vi "FL_Calculate_phi_theta_etc.vi"(5 "Mouse face dir. swap":bool, 6 "x1-x2":sgl, 7 "R from center":sgl, 8 "y1-y2":sgl, 9 "Mouse Yc":sgl, 10 "MouseXc":sgl, 11 "sin(a)":sgl) -> (3 "Output data cluster":T1)   [LabVIEW 2018, in "Tracker.lvlib"]
uses:
  Tracker.lvlib
panel:
  out "Mouse rot. angle":sgl
  out "from center towards mouse":sgl
  out "Rel Y":sgl
  out "Rel X":sgl
  out "mouse wall angle":sgl
  out "phi":sgl
  out "Cage rotation against mouse":sgl
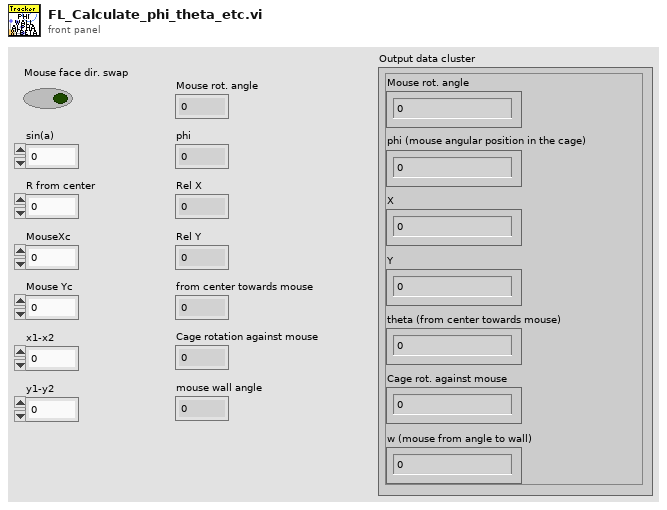
[diagram p1: front panel]
types:
  T1 = cluster{"Mouse rot. angle":sgl, "phi (mouse angular position in the cage)":dbl, "X":dbl, "Y":dbl, "theta (from center towards mouse)":dbl, "Cage rot. against mouse":sgl, "w (mouse from angle to wall)":dbl}
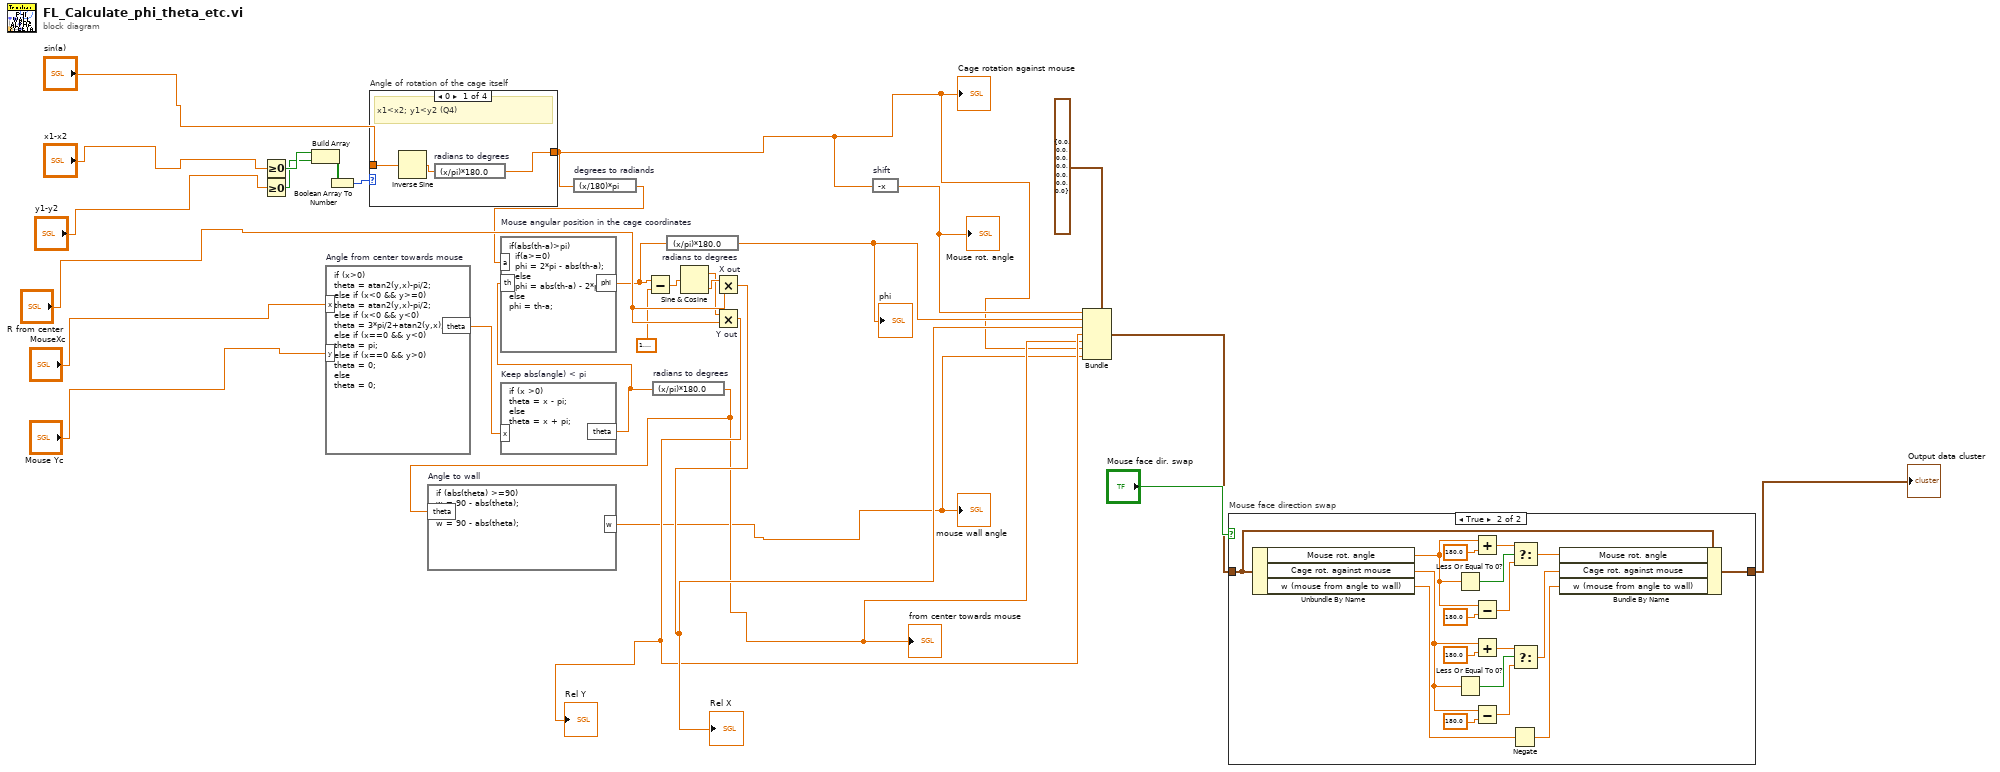
[diagram p0: block diagram]
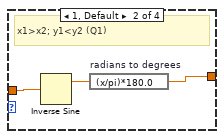
[diagram p3: hidden frame]
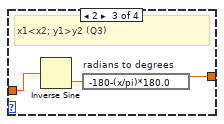
[diagram p4: hidden frame]
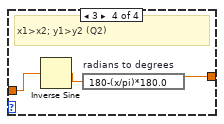
[diagram p5: hidden frame]
diagram:
  n1 = Greater Or Equal To 0?(x="x1-x2") -> (x >= 0?=w23:bool)
  n2 = Greater Or Equal To 0?(x="y1-y2") -> (x >= 0?=w22:bool)
  n3 = Build Array(w23, w22) -> (w21:bool[])
  n4 = formula code="if (x>0)\ntheta = atan2(y,x)-pi/2;\nelse if (x<0 && y>=0)\ntheta = atan2(y,x)-pi/2;\nelse if (x<0 && y<0)\ntheta = 3*pi/2+atan2(y,x);\nelse if (x==0 && y<0)\ntheta = pi;\nelse if (x==0 && y>0)\ntheta = 0;\nelse\ntheta = 0;" "Angle from center towards mouse"("x"="MouseXc", "y"="Mouse Yc") -> ("theta"=w19:dbl)
  n5 = Boolean Array To Number(Boolean array=w21) -> (number=w20:u32)
  n6 = case "Angle of rotation of the cage itself" shown="0" w20 {
    tunnel: "sin(a)" -> [w31 w34 w37 w40]
    tunnel: [w30 w33 w36 w39] -> w6
    frame 0 {
      # "x1<x2; y1<y2 (Q4)"
      n7 = Inverse Sine(1:w31) -> (0:w32:sgl)
      n8 = expression code="(x/pi)*180.0" "radians to degrees"(w32) -> (w30:sgl)
    }
    frame 1, Default {
      # "x1>x2; y1<y2 (Q1)"
      n9 = Inverse Sine(1:w34) -> (0:w35:sgl)
      n10 = expression code="(x/pi)*180.0" "radians to degrees"(w35) -> (w33:sgl)
    }
    frame 2 {
      # "x1<x2; y1>y2 (Q3)"
      n11 = Inverse Sine(1:w37) -> (0:w38:sgl)
      n12 = expression code="-180-(x/pi)*180.0" "radians to degrees"(w38) -> (w36:sgl)
    }
    frame 3 {
      # "x1>x2; y1>y2 (Q2)"
      n13 = Inverse Sine(1:w40) -> (0:w41:sgl)
      n14 = expression code="180-(x/pi)*180.0" "radians to degrees"(w41) -> (w39:sgl)
    }
  }
  "Cage rotation against mouse" <- w6
  n15 = formula code="if (x >0)\ntheta = x - pi;\nelse\ntheta = x + pi;" "Keep abs(angle) < pi"("x"=w19) -> ("theta"=w16:dbl)
  n16 = expression code="(x/180)*pi" "degrees to radiands"(w6) -> (w15:sgl)
  n17 = formula code="if(abs(th-a)>pi)\n  if(a>=0)\n  phi = 2*pi - abs(th-a);\n  else\n  phi = abs(th-a) - 2*pi;\nelse\nphi = th-a;" "Mouse angular position in the cage coordinates"("th"=w16, "a"=w15) -> ("phi"=w13:dbl)
  n18 = Subtract(x=w13, y=1.5707963267948966) -> (x-y=w14:dbl)
  n19 = expression code="(x/pi)*180.0" "radians to degrees"(w16) -> (w7:dbl)
  "from center towards mouse" <- w7
  n20 = formula code="if (abs(theta) >=90)\nw = 90 - abs(theta);\nelse\nw = 90 - abs(theta);" "Angle to wall"("theta"=w7) -> ("w"=w1:dbl)
  "mouse wall angle" <- w1
  n21 = expression code="(x/pi)*180.0" "radians to degrees"(w13) -> (w10:dbl)
  "phi" <- w10
  n22 = Sine & Cosine(0:w14) -> (1:w17:dbl, 2:w18:dbl)
  n23 = Multiply "X out"(x=w18, y="R from center") -> (x*y=w9:dbl)
  "Rel X" <- w9
  n24 = Multiply "Y out"(x=w17, y="R from center") -> (x*y=w8:dbl)
  "Rel Y" <- w8
  n25 = expression code="-x" "shift"(w6) -> (w11:sgl)
  "Mouse rot. angle" <- w11
  n26 = Bundle(cluster=T1 {"Mouse rot. angle"=0.0, "phi (mouse angular position in the cage)"=0.0, "X"=0.0, "Y"=0.0, "theta (from center towards mouse)"=0.0, "Cage rot. against mouse"=0.0, "w (mouse from angle to wall)"=0.0} ("Output data cluster 2"), "Mouse rot. angle"=w11, "phi (mouse angular position in the cage)"=w10, "X"=w9, "Y"=w8, "theta (from center towards mouse)"=w7, "Cage rot. against mouse"=w6, "w (mouse from angle to wall)"=w1) -> (w2:T1)
  n27 = case "Mouse face direction swap" shown="True" "Mouse face dir. swap" {
    tunnel: [w42 w54] -> w3
    tunnel: w2 -> [w42 w55]
    frame False {
    }
    frame True {
      n28 = Unbundle By Name(w55) -> ("Mouse rot. angle"=w53:sgl, "Cage rot. against mouse"=w46:sgl, "w (mouse from angle to wall)"=w44:dbl)
      n29 = Less Or Equal To 0?(x=w53) -> (x <= 0?=w60:bool)
      n30 = Less Or Equal To 0?(x=w46) -> (x <= 0?=w47:bool)
      n31 = Add(x=w53, y=sgl 180.0) -> (x+y=w57:sgl)
      n32 = Subtract(x=w53, y=sgl 180.0) -> (x-y=w59:sgl)
      n33 = Add(x=w46, y=sgl 180.0) -> (x+y=w50:sgl)
      n34 = Subtract(x=w46, y=sgl 180.0) -> (x-y=w48:sgl)
      n35 = Negate(x=w44) -> (-x=w43:dbl)
      n36 = Select(t=w57, s=w60, f=w59) -> (s? t:f=w52:sgl)
      n37 = Select(t=w50, s=w47, f=w48) -> (s? t:f=w45:sgl)
      n38 = Bundle By Name(cluster=w55, "Mouse rot. angle"=w52, "Cage rot. against mouse"=w45, "w (mouse from angle to wall)"=w43) -> (w54:T1)
    }
  }
  "Output data cluster" <- w3
